vi "Barcode_Reader_Base_SoftFP.vi"(0 "reference in":refnum<class "Barcode_Reader_Base.lvclass">, 5 "error in (no error)":errorcluster) -> (14 "reference out":refnum<class "Barcode_Reader_Base.lvclass">, 19 "error out":errorcluster)   [LabVIEW 2022 SP3, in "Barcode_Reader_Base.lvlib" / "Barcode_Reader_Base.lvclass"]
uses:
  Barcode_Reader_Base.lvclass
  Components/ViPER.lvlibp/ViPER.lvclass
  C:/Projects/Medulla/ViPER/Examples/Flux_Capacitor_Tester/Components/ViPER.lvlibp/ViPER.lvclass
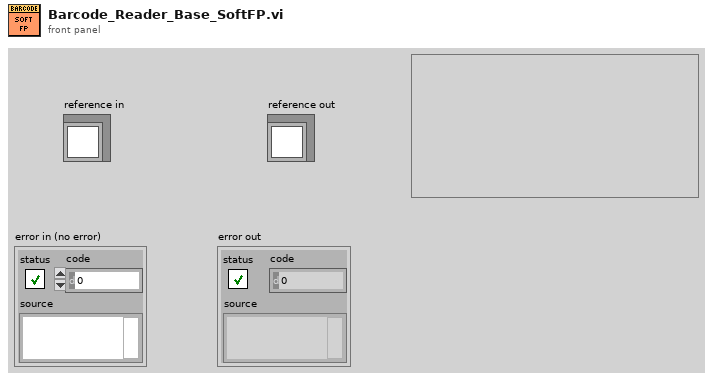
[diagram p1: front panel]
types:
  T1 = enum32{"Invalid", "Standard", "Closed", "Hidden", "Minimized", "Maximized"}
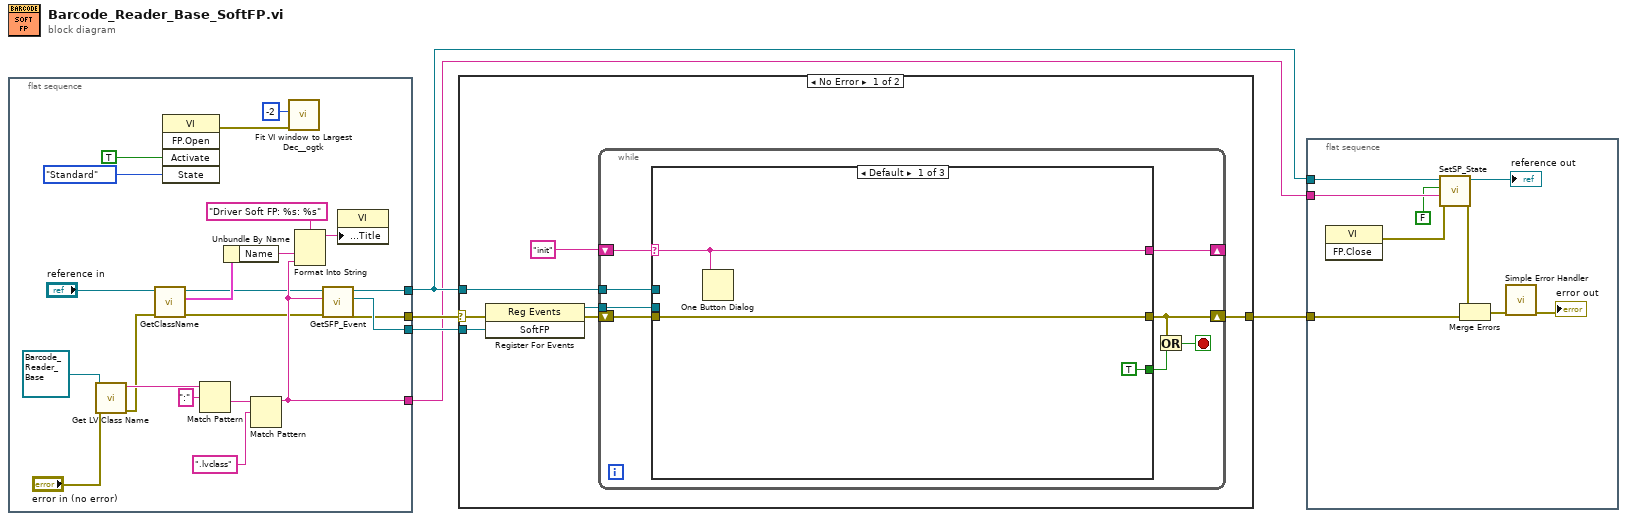
[diagram p0: block diagram]
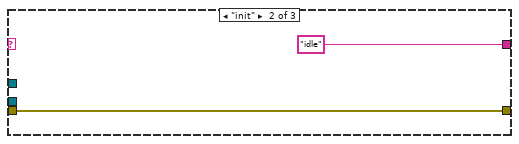
[diagram p2: hidden frame]
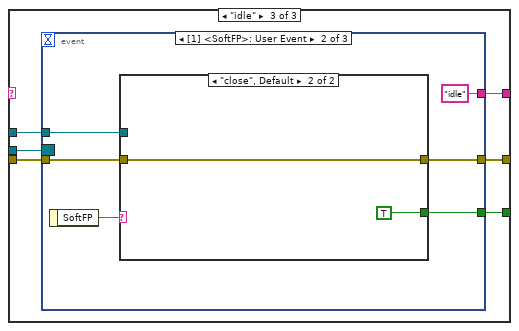
[diagram p3: hidden frame]
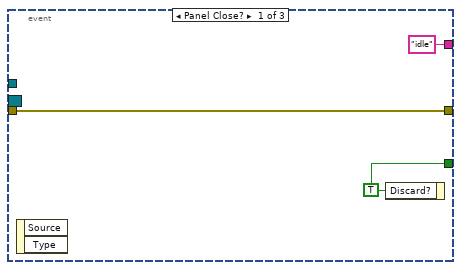
[diagram p4: hidden frame]
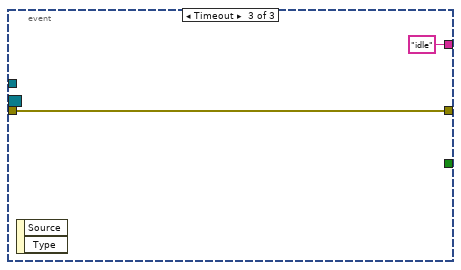
[diagram p6: hidden frame]
diagram:
  n1 = flat-sequence {
    tunnel: [w21] -> w5
    tunnel: [w20] -> w2
    tunnel: [w24] -> w3
    tunnel: [w11] -> w1
    frame #0 {
      n2 = call <vilib>:"Get LV Class Name.vi"("error in (no error)"="error in (no error)", "object"=refnum<class "Barcode_Reader_Base.lvclass"> refnum ("reference")) -> ("error out"=w10:errorcluster, "class name"=w16:string)  [unwired: 8 in]
      n3 = call "GetClassName.vi"("error in (no error)"=w10, "reference in"="reference in") -> ("error out"=w9:errorcluster, "Details"=w8:cluster{"Name":string, "Class":string}, "reference out"=w6:refnum<class "Barcode_Reader_Base.lvclass">)  [unwired: 7 in]
      n4 = invoke class="VI" method="FP.Open"("Activate"=TRUE ("Activate?"), "State"=T1."Standard") -> (error out=w18:errorcluster)  [unwired: 3 in, 4 out]
      n5 = Match Pattern(string=w16, regular expression=":") -> (after substring=w14:string)  [unwired: 1 in, 3 out]
      n6 = Unbundle By Name(w8) -> ("Name"=w19:string)
      n7 = Match Pattern(string=w14, regular expression=".lvclass") -> (before substring=w11:string)  [unwired: 1 in, 3 out]
      n8 = call <userlib>:"Fit VI window to Largest Dec__ogtk.vi"("error in (no error)"=w18, "border spacing (2 px)"=-2) -> ()  [unwired: 4 in, 2 out]
      n9 = Format Into String(format string="Driver Soft FP: %s: %s", w19, w11) -> (resulting string=w23:string)  [unwired: 2 in, 1 out]
      n10 = call-dynamic "GetSFP_Event.vi"("error in (no error)"=w9, "Ancestor"=w11, "reference in"=w6) -> ("error out"=w21:errorcluster, "SoftFP"=w24:refnum<user-event>, "reference out"=w20:refnum<class "Barcode_Reader_Base.lvclass">)  [unwired: 6 in]
      n11 = property class="VI"("Front Panel.Title"=w23) -> ()  [unwired: 2 in, 2 out]
    }
  }
  n12 = case shown="No Error" w5 {
    selector: w5 -> [w32 w68]
    tunnel: [w28 w68] -> w4
    tunnel: w2 -> [w29 _]
    tunnel: w3 -> [w34 _]
    frame No Error {
      n13 = register-events(error in=w32, w34) -> (reference out=w33:refnum<event-registration>, error out=w31:errorcluster)  [unwired: 1 in]
      n14 = while {
        shift-right: [w39] -> w28
        shift-left: w31 -> [w42]
        tunnel: w33 -> [w41]
        tunnel: w29 -> [w40]
        shift-right: [w35] -> _
        shift-left: "init" -> [w36]
        stop <- w38 stop-if-true
        n15 = case shown="Default" w36 {
          selector: w36 -> [w43 _ _]
          tunnel: w42 -> [w44 w46 w53]
          tunnel: w41 -> [_ _ w52]
          tunnel: w40 -> [_ _ w51]
          tunnel: [w44 w46 w50] -> w39
          tunnel: [TRUE ("Discard?") _ w49] -> w37
          tunnel: [w43 "idle" w48] -> w35
          frame Default {
            n16 = One Button Dialog(message=w43) -> ()  [unwired: 1 in, 1 out]
          }
          frame "init" {
          }
          frame "idle" {
            n17 = event shown="[1] <SoftFP>: User Event" {
              selector: w52 -> [_ _ _]
              dyn-events: _ -> [_ _ _]
              timeout: _ -> [_ _ _]
              tunnel: w53 -> [w56 w62 w67]
              tunnel: [w56 w60 w67] -> w50
              tunnel: [w55 w59 _] -> w49
              tunnel: w51 -> [_ w57 _]
              tunnel: ["idle" "idle" "idle"] -> w48
              event Panel Close? {
                w55 = TRUE ("Discard?")
                n18 = event-data() -> ()  [unwired: 1 in, 2 out]
                n19 = event-data("Discard?"=w55) -> ()  [unwired: 1 in, 1 out]
              }
              event User Event {
                n20 = event-data() -> ("SoftFP"=w61:string)  [unwired: 1 in]
                n21 = case shown="\"close\", Default" w61 {
                  tunnel: w62 -> [w63 w65]
                  tunnel: [w63 w65] -> w60
                  tunnel: [_ TRUE ("Discard?")] -> w59
                  tunnel: w57 -> [_ _]
                  frame "UpdateUI" {
                  }
                  frame "close", Default {
                  }
                }
              }
              event Timeout {
                n22 = event-data() -> ()  [unwired: 1 in, 2 out]
              }
            }
          }
        }
        n23 = Or(x=w39, y=w37) -> (x .or. y?=w38:bool)
      }
    }
    frame Error {
    }
  }
  n24 = flat-sequence {
    tunnel: w4 -> [w75]
    tunnel: w2 -> [w70]
    tunnel: w1 -> [w72]
    frame #0 {
      n25 = invoke class="VI" method="FP.Close"() -> (error out=w74:errorcluster)  [unwired: 3 in, 2 out]
      n26 = call "SetSP_State.vi"("error in (no error)"=w74, "Ancestor"=w72, "SP Open"=FALSE, "reference in"=w70) -> ("error out"=w73:errorcluster, "reference out"=→"reference out":refnum<class "Barcode_Reader_Base.lvclass">)  [unwired: 6 in]
      n27 = Merge Errors(w73, w75) -> (w77:errorcluster)
      n28 = call <vilib>:"Simple Error Handler.vi"("error in (no error)"=w77) -> ("error out"=→"error out":errorcluster)  [unwired: 4 in, 4 out]
    }
  }
